vi "Send ACQ Notification.vi"(8 "error in (no error)":errorcluster, 10 "1 Sample":T1, 11 "ACQ Data Notifier in":refnum<notifier>) -> (0 "error out":errorcluster, 3 "ACQ Data Notifier out":refnum<notifier>)   [LabVIEW 2014, in "WINFAS 2 Data Queue.lvlib"]
uses:
  Acquisition Data 1 Sample Cluster.ctl
  WINFAS 2 Data Queue.lvlib
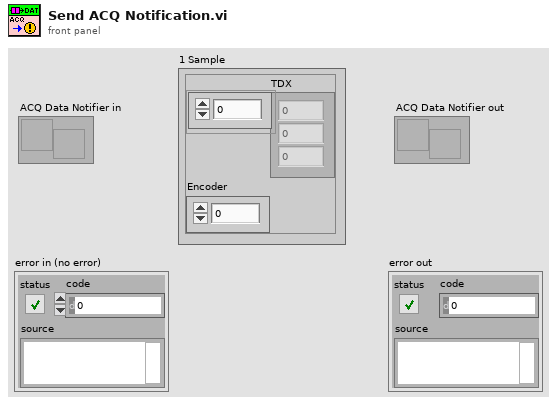
[diagram p1: front panel]
types:
  T1 = typedef "WINFAS 2 Data Queue.lvlib/Acquisition Data 1 Sample Cluster.ctl" = cluster{"TDX":sgl[], "Encoder":sgl}
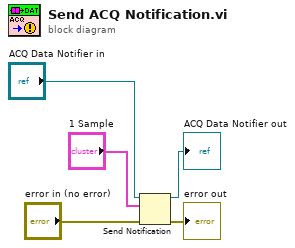
[diagram p0: block diagram]
diagram:
  n1 = Send Notification(notification="1 Sample", notifier="ACQ Data Notifier in", error in (no error)="error in (no error)") -> (notifier out=→"ACQ Data Notifier out":refnum<notifier>, error out=→"error out":errorcluster)
